vi "Paint_figure.vi"() -> ()   [LabVIEW 2013]
panel:
  out "Array":dbl[](array[numeric])
  in  "OK Button":bool
  out "2D Picture":picture
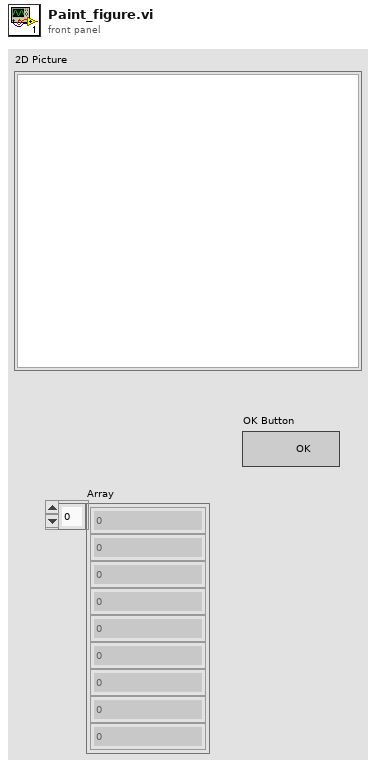
[diagram p1: front panel]
types:
  T1 = typedef "LVPoint32TypeDef.ctl" = cluster{"Horizontal":i32, "Vertical":i32}
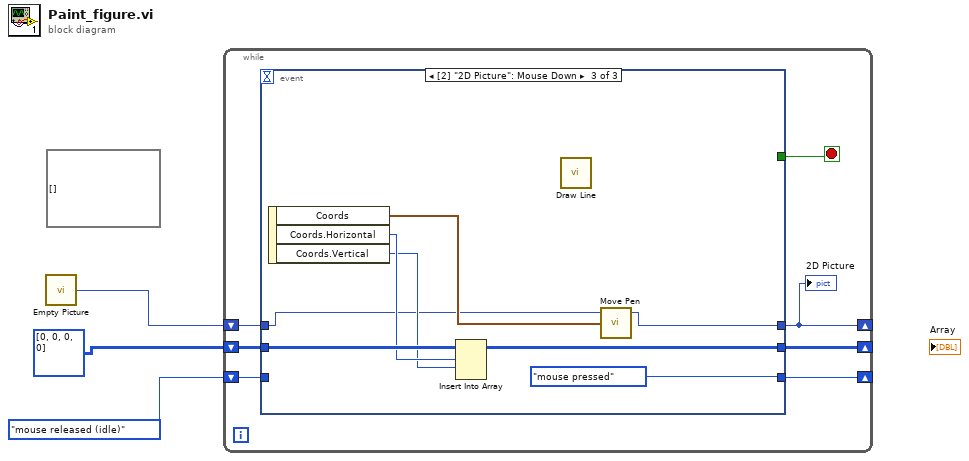
[diagram p0: block diagram]
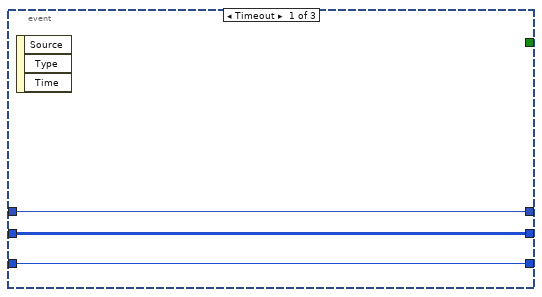
[diagram p2: hidden frame]
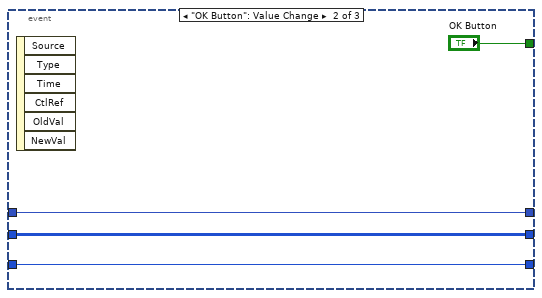
[diagram p3: hidden frame]
diagram:
  (unwired) void[] []
  n1 = call "Empty Picture"() -> ("empty picture"=w2:picture)
  n2 = while {
    shift-right: [w5] -> _
    shift-left: enum16{"mouse released (idle)", "mouse pressed"}."mouse released (idle)" -> [w9]
    shift-right: [w7] -> _
    shift-left: w2 -> [w8]
    shift-right: [w6] -> _
    shift-left: i32[][] [[0, 0], [0, 0]] -> [w10]
    stop <- w4 stop-if-true
    n3 = event shown="[2] \"2D Picture\": Mouse Down" {
      selector: _ -> [_ _ _]
      dyn-events: _ -> [_ _ _]
      timeout: _ -> [_ _ _]
      tunnel: w10 -> [w12 w16 w24]
      tunnel: w9 -> [w11 w14 _]
      tunnel: w8 -> [w13 w15 w19]
      tunnel: [w13 w15 w18] -> w7
      tunnel: [w12 w16 w21] -> w6
      tunnel: [w11 w14 enum16{"mouse released (idle)", "mouse pressed"}."mouse pressed"] -> w5
      tunnel: [_ "OK Button" _] -> w4
      event Timeout {
        n4 = event-data() -> ()  [unwired: 1 in, 3 out]
      }
      event "OK Button": Value Change {
        n5 = event-data() -> ()  [unwired: 1 in, 6 out]
      }
      event "2D Picture": Mouse Down {
        n6 = event-data() -> ("Coords"=w20:T1, "Coords.Horizontal"=w23:i32, "Coords.Vertical"=w22:i32)  [unwired: 1 in]
        n7 = Insert Into Array(array=w24, index (row)=w23, index (col)=w22) -> (w21:i32[][])  [unwired: 1 in]
        n8 = call <vilib>:"Draw Line.vi"() -> ()  [unwired: 9 in, 1 out]
        n9 = call <vilib>:"Move Pen.vi"("new position"=w20, "picture"=w19) -> ("new picture"=w18:picture)  [unwired: 3 in]
      }
    }
    "2D Picture" <- w7
  }
